vi "h5_1D_DBL.vi"(6 "Attributes":variant, 7 "TYPE":string, 8 "error in (no error)":errorcluster, 9 "1D DBL":dbl[](array[numeric]), 10 "SQUID":string, 11 "H5":path[](array[path])) -> (0 "error out":errorcluster, 2 "Exists":bool)   [LabVIEW 2013]
uses:
  <vilib>/addons/h5labview2/file/H5Fmode.ctl
  <vilib>/addons/h5labview2/base/lib_path.vi
  <vilib>/addons/h5labview2/base/H5Equery.vi
  <vilib>/addons/h5labview2/dataset/H5Dwrite.llb/H5Dwrite.xnode
  <vilib>/addons/h5labview2/base/hid_t.ctl
  <vilib>/addons/h5labview2/file/H5F.lvlib
  <vilib>/addons/h5labview2/dataset/H5D.lvlib
  <vilib>/addons/h5labview2/group/H5G.lvlib
  <vilib>/addons/h5labview2/space/H5S.lvlib
  <vilib>/addons/h5labview2/attrib/H5A.lvlib
panel:
  out "error out 2":errorcluster
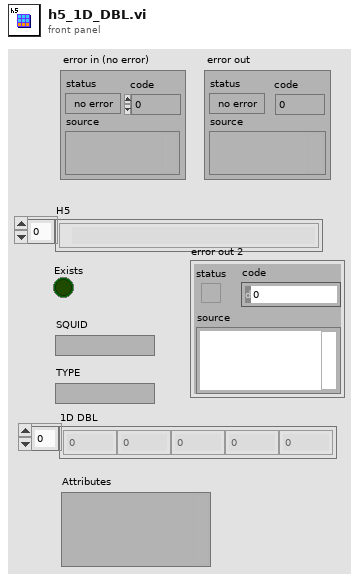
[diagram p1: front panel]
types:
  T1 = typedef "Semaphore RefNum" = refnum<k1>
  T2 = typedef "H5F.lvlib/H5Fmode.ctl" = enum16{"read-only", "read-write", "overwrite", "create new", "open or create"}
  T3 = typedef "hid_t.ctl" = i32
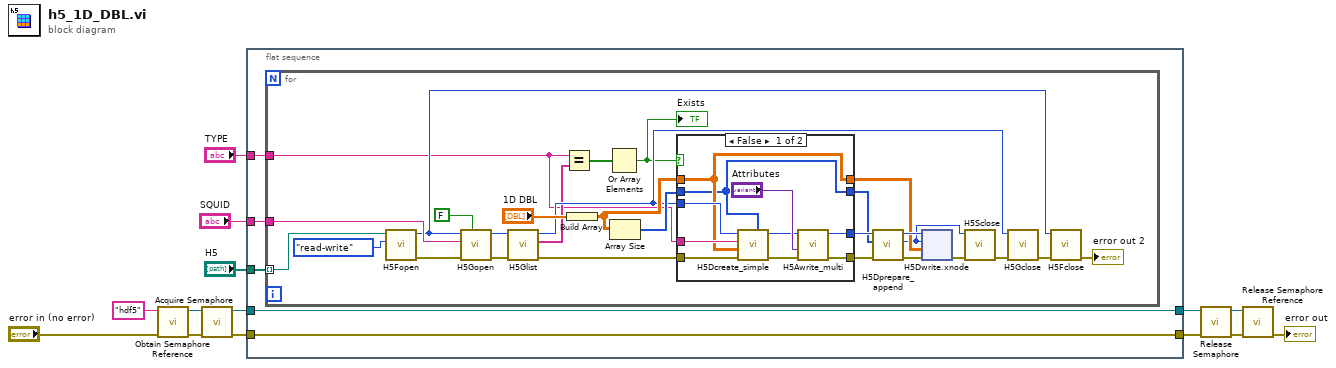
[diagram p0: block diagram]
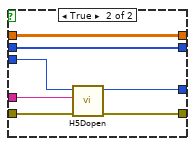
[diagram p2: hidden frame]
diagram:
  n1 = call <vilib>:"Obtain Semaphore Reference.vi"("error in (no error)"="error in (no error)", "name (unnamed)"="hdf5") -> ("error out"=w13:errorcluster, "semaphore"=w14:T1)  [unwired: 3 in, 1 out]
  n2 = call <vilib>:"Acquire Semaphore.vi"("error in (no error)"=w13, "semaphore"=w14) -> ("error out"=w7:errorcluster, "semaphore out"=w6:T1)  [unwired: 3 in, 1 out]
  n3 = flat-sequence {
    tunnel: [w19] -> w8
    tunnel: w7 -> [w19]
    tunnel: w6 -> [w18]
    tunnel: [w18] -> w5
    tunnel: "H5" -> [w17]
    tunnel: "SQUID" -> [w16]
    tunnel: "TYPE" -> [w15]
    frame #0 {
      n4 = for {
        tunnel: w17 -> [w30] mode=indexing
        tunnel: w16 -> [w31]
        tunnel: w15 -> [w22]
        n5 = call <vilib>:"H5Fopen.vi"("mode (read-only)"=H5Fmode."read-write", "path"=w30) -> ("error out"=w29:errorcluster, "ref out"=w28:T3)  [unwired: 8 in]
        n6 = call <vilib>:"H5Gopen.vi"("create? (F)"=FALSE, "error in (no error)"=w29, "name"=w31, "ref in"=w28) -> ("error out"=w26:errorcluster, "group out"=w27:T3)  [unwired: 6 in]
        n7 = call <vilib>:"H5Glist.vi"("error in (no error)"=w26, "ref in"=w27) -> ("error out"=w25:errorcluster, "names"=w23:string[], "ref out"=w24:T3)  [unwired: 6 in, 1 out]
        n8 = Equal?(x=w22, y=w23) -> (x = y?=w21:bool[])
        n9 = Build Array("1D DBL") -> (w40:dbl[][])
        n10 = Or Array Elements(Boolean array=w21) -> (logical OR=w20:bool)
        "Exists" <- w20
        n11 = Array Size(array=w40) -> (size(s)=w41:i32[])
        n12 = case shown="False" w20 {
          tunnel: w25 -> [w75 w80]
          tunnel: w40 -> [w72 w82]
          tunnel: w24 -> [w74 w77]
          tunnel: w22 -> [w73 w78]
          tunnel: [w68 w79] -> w46
          tunnel: [w69 w76] -> w45
          tunnel: w41 -> [w71 w81]
          tunnel: [w72 w82] -> w37
          tunnel: [w71 w81] -> w39
          frame False {
            n13 = call <vilib>:"H5Dcreate_simple.vi"("chunk size"=w71, "error in (no error)"=w75, "type in"=w72, "name"=w73, "ref in"=w74) -> ("error out"=w67:errorcluster, "dset out"=w66:T3)  [unwired: 5 in]
            n14 = call <vilib>:"H5Awrite_multi.vi"("error in (no error)"=w67, "variant in"="Attributes", "ref in"=w66) -> ("error out"=w68:errorcluster, "ref out"=w69:T3)  [unwired: 7 in]
          }
          frame True {
            n15 = call <vilib>:"H5Dopen.vi"("error in (no error)"=w80, "name"=w78, "loc in"=w77) -> ("error out"=w79:errorcluster, "dset out"=w76:T3)  [unwired: 7 in]
          }
        }
        n16 = call <vilib>:"H5Dprepare_append.vi"("error in (no error)"=w46, "append dims"=w39, "dset in"=w45) -> ("error out"=w44:errorcluster, "space out"=w36:T3, "dset out"=w38:T3)  [unwired: 6 in]
        n17 = xnode "H5Dwrite.xnode"("error in (no error)"=w44, "data"=w37, "file space"=w36, "ref in"=w38) -> ("error out"=w43:errorcluster)  [unwired: 3 in, 2 out]
        n18 = call <vilib>:"H5Sclose.vi"("error in (no error)"=w43, "space in"=w36) -> ("error out"=w34:errorcluster)  [unwired: 9 in]
        n19 = call <vilib>:"H5Gclose.vi"("error in (no error)"=w34, "group in"=w24) -> ("error out"=w32:errorcluster)  [unwired: 9 in]
        n20 = call <vilib>:"H5Fclose.vi"("error in (no error)"=w32, "ref"=w28) -> ("error out"=→"error out 2":errorcluster)  [unwired: 9 in]
      }
    }
  }
  n21 = call <vilib>:"Release Semaphore.vi"("error in (no error)"=w8, "semaphore"=w5) -> ("error out"=w9:errorcluster, "semaphore out"=w10:T1)  [unwired: 4 in]
  n22 = call <vilib>:"Release Semaphore Reference.vi"("error in (no error)"=w9, "semaphore"=w10) -> ("error out"=→"error out":errorcluster)  [unwired: 8 in, 1 out]
